vi "Parse OUTCAR.vi"(8 "error in (no error)":errorcluster, 11 "OUTCAR File":path) -> (0 "error out":errorcluster, 2 "Relaxation Time":timestamp, 3 "Calc Time (Hrs)":dbl)   [LabVIEW 2010]
uses:
  <vilib>/Utility/error.llb/whitespace.ctl
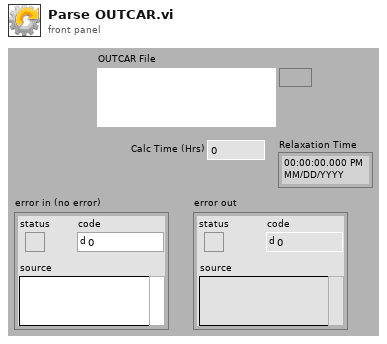
[diagram p1: front panel]
types:
  T1 = cluster{"fraction":dbl, "second":i32, "minute":i32, "hour":i32, "day of month":i32, "month":i32, "year":i32, "day of week":i32, "day of year":i32, "is DST":i32}
  T2 = typedef "whitespace.ctl" = u16
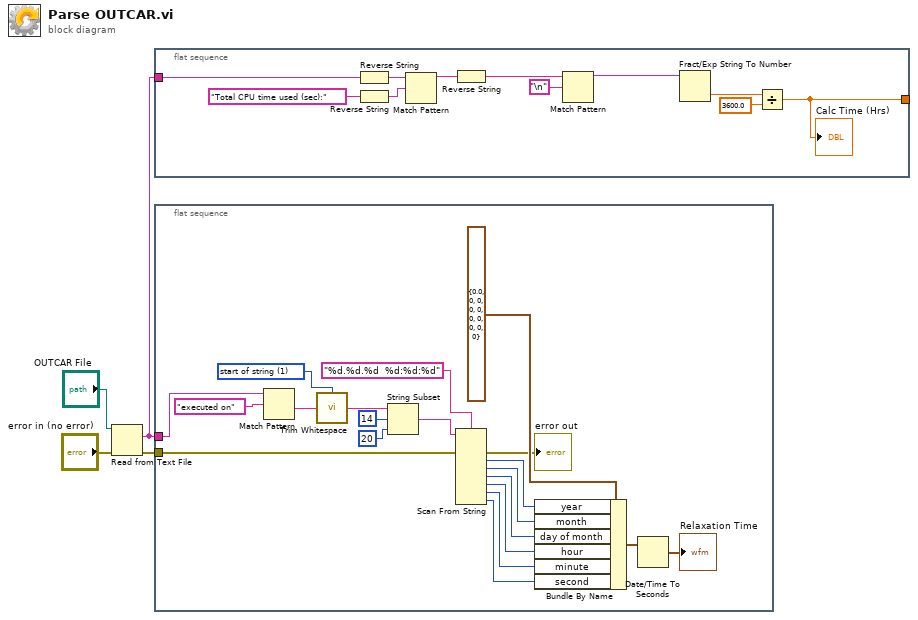
[diagram p0: block diagram]
diagram:
  n1 = Read from Text File(file (use dialog)="OUTCAR File", error in="error in (no error)") -> (text=w2:string, error out=w1:errorcluster)  [unwired: 2 in, 2 out]
  n2 = flat-sequence {
    tunnel: w2 -> [w15]
    tunnel: [w5] -> _
    frame #0 {
      n3 = Reverse String(1:w15) -> (0:w14:string)
      n4 = Reverse String(1:"Total CPU time used (sec):" ("regular expression")) -> (0:w12:string)
      n5 = Match Pattern(string=w14, regular expression=w12) -> (before substring=w9:string)  [unwired: 1 in, 3 out]
      n6 = Reverse String(1:w9) -> (0:w11:string)
      n7 = Match Pattern(string=w11, regular expression="\n") -> (before substring=w8:string)  [unwired: 1 in, 3 out]
      n8 = Fract/Exp String To Number(string=w8) -> (number=w7:dbl)  [unwired: 3 in, 1 out]
      n9 = Divide(x=w7, y=3600.0) -> (x/y=w5:dbl)
      "Calc Time (Hrs)" <- w5
    }
  }
  n10 = flat-sequence {
    tunnel: w2 -> [w35]
    tunnel: w1 -> [w17]
    frame #0 {
      w22 = T2 1 items=["both", "start of string", "end of string"] ("location (both)")
      n11 = Match Pattern(string=w35, regular expression="executed on") -> (after substring=w21:string)  [unwired: 1 in, 3 out]
      n12 = call <vilib>:"Trim Whitespace.vi"("string"=w21, "location (both)"=w22) -> ("trimmed string"=w20:string)
      n13 = String Subset(string=w20, offset (0)=14, length (rest)=20 ("length (rest)")) -> (substring=w19:string)
      n14 = Scan From String(format string="%d.%d.%d  %d:%d:%d", input string=w19, error in=w17) -> (error out=→"error out":errorcluster, output 1=w29:i32, output 2=w28:i32, output 3=w27:i32, output 4=w26:i32, output 5=w25:i32, output 6=w24:i32)  [unwired: 7 in, 2 out]
      n15 = Bundle By Name(cluster=T1 {"fraction"=0.0, "second"=0, "minute"=0, "hour"=0, "day of month"=0, "month"=0, "year"=0, "day of week"=0, "day of year"=0, "is DST"=0} ("new date time rec"), "year"=w29, "month"=w28, "day of month"=w27, "hour"=w26, "minute"=w25, "second"=w24) -> (w30:T1)
      n16 = Date/Time To Seconds(2:w30) -> (0:→"Relaxation Time":timestamp)  [unwired: 1 in]
    }
  }
